vi "Evaluate SW Version Response.vi"(1 "String In":string) -> (0 "Test OK":bool)   [LabVIEW 2022 SP3]
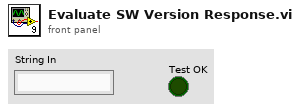
[diagram p1: front panel]
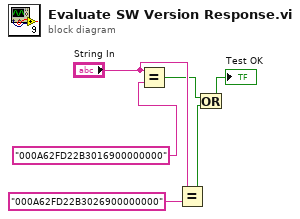
[diagram p0: block diagram]
diagram:
  n1 = Equal?(x="String In", y="000A62FD22B3016900000000") -> (x = y?=w3:bool)
  n2 = Equal?(x="String In", y="000A62FD22B3026900000000") -> (x = y?=w2:bool)
  n3 = Or(x=w3, y=w2) -> (x .or. y?=→"Test OK":bool)
